vi "Check ElapsedTime.vi"(8 "error in":errorcluster, 11 "Switch in":refnum<class "Switch.lvclass">) -> (0 "error out":errorcluster, 1 "LastSwitch":timestamp, 2 "Cycle Switch?":bool, 3 "Switch out":refnum<class "Switch.lvclass">)   [LabVIEW 2014, in "Switch.lvclass"]
doc: "Check to see if the maximum time has elapsed for a particular state. If so, and the value of the maxElapsedTime is > 0, change the state."
uses:
  Switch.lvclass
  Switch.lvclass/Switch.ctl
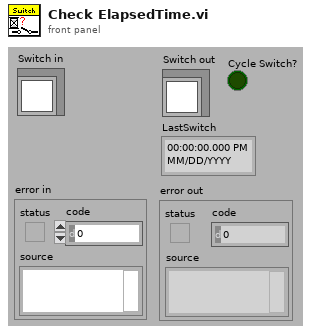
[diagram p1: front panel]
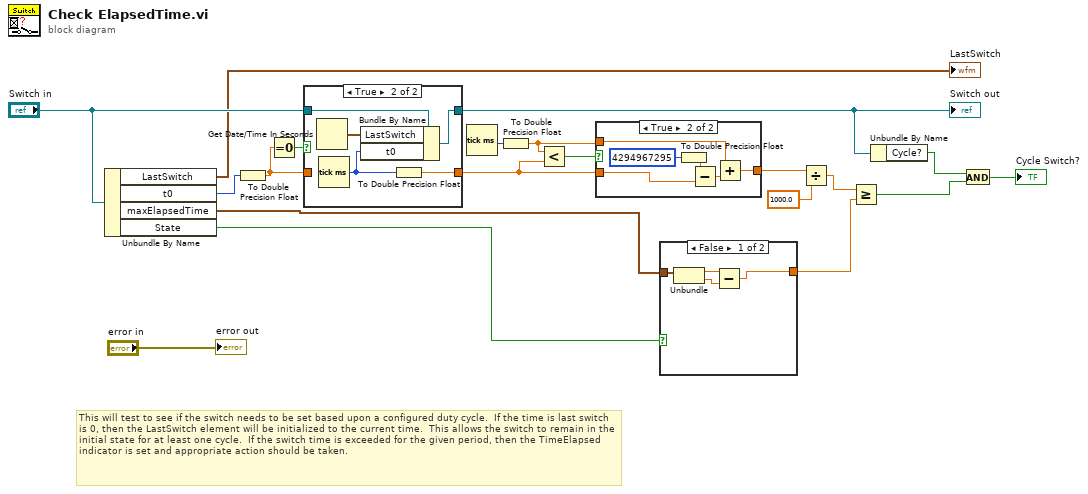
[diagram p0: block diagram]
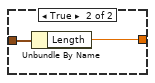
[diagram p2: hidden frame]
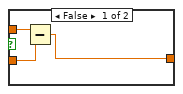
[diagram p3: hidden frame]
diagram:
  # "This will test to see if the switch needs to be set based upon a configured duty cycle.  If the time is last switch is 0, then the LastSwitch element will be initialized to the current time.  This allows the switch to remain in the initial state for at least one cycle.  If the switch time is exceeded for the given period, then the TimeElapsed indicator is set and appropriate action should be taken."
  n1 = Unbundle By Name("Switch in") -> ("LastSwitch"=→"LastSwitch":timestamp, "t0"=w13:u32, "maxElapsedTime"=w7:cluster{"Period":sgl, "Length":sgl}, "State"=w8:bool)
  n2 = To Double Precision Float(number=w13) -> (double precision float=w16:dbl)
  n3 = Equal To 0?(x=w16) -> (x = 0?=w17:bool)
  n4 = case shown="True" w17 {
    tunnel: w16 -> [w22 _]
    tunnel: "Switch in" -> [w21 w27]
    tunnel: [w22 w24] -> w10
    tunnel: [w21 w26] -> w4
    frame False {
    }
    frame True {
      n5 = Get Date/Time In Seconds() -> (seconds since 1Jan1904=w25:timestamp)
      n6 = Tick Count (ms)() -> (millisecond timer value=w23:u32)
      n7 = Bundle By Name(cluster=w27, "LastSwitch"=w25, "t0"=w23) -> (w26:refnum<class "Switch.lvclass">)
      n8 = To Double Precision Float(number=w23) -> (double precision float=w24:dbl)
    }
  }
  "Switch out" <- w4
  n9 = Tick Count (ms)() -> (millisecond timer value=w15:u32)
  n10 = To Double Precision Float(number=w15) -> (double precision float=w11:dbl)
  n11 = Less?(x=w11, y=w10) -> (x < y?=w12:bool)
  n12 = case shown="True" w12 {
    tunnel: w11 -> [w30 w31]
    tunnel: w10 -> [w29 w33]
    tunnel: [w28 w34] -> w9
    frame False {
      n13 = Subtract(x=w30, y=w29) -> (x-y=w28:dbl)
    }
    frame True {
      n14 = To Double Precision Float(number=u32 4294967295 ("millisecond timer value")) -> (double precision float=w35:dbl)
      n15 = Subtract(x=w35, y=w33) -> (x-y=w32:dbl)
      n16 = Add(x=w31, y=w32) -> (x+y=w34:dbl)
    }
  }
  n17 = case shown="False" w8 {
    tunnel: w7 -> [w40 w42]
    tunnel: [w37 w41] -> w5
    frame False {
      n18 = Unbundle(w40) -> ("Period"=w39:sgl, "Length"=w38:sgl)
      n19 = Subtract(x=w39, y=w38) -> (x-y=w37:sgl)
    }
    frame True {
      n20 = Unbundle By Name(w42) -> ("Length"=w41:sgl)
    }
  }
  n21 = Divide(x=w9, y=1000.0) -> (x/y=w6:dbl)
  n22 = Greater Or Equal?(x=w6, y=w5) -> (x >= y?=w2:bool)
  n23 = Unbundle By Name(w4) -> ("Cycle?"=w3:bool)
  n24 = And(x=w3, y=w2) -> (x .and. y?=→"Cycle Switch?":bool)
  "error out" <- "error in"
